vi "Deep Copy.vi"(8 "error in (no error)":errorcluster, 10 "Copy Actor In":refnum<class "System Actor.lvclass">, 11 "Root Actor in":refnum<class "Root Actor.lvclass">) -> (0 "error out":errorcluster, 2 "Coppied Actor Out":refnum<class "System Actor.lvclass">, 3 "Root Actor out":refnum<class "Root Actor.lvclass">)   [LabVIEW 2024, in "Root Actor.lvclass"]
uses:
  Root Actor.lvclass
  C:/Users/iio/Desktop/Bussiness/Tricorn Re/Madelbrot 4.0/General Library/Ancestor Class/Actor/System Actor/System Actor.lvclass
  System Actor/System Actor.lvclass
  Root Actor.lvclass/Root Actor.ctl
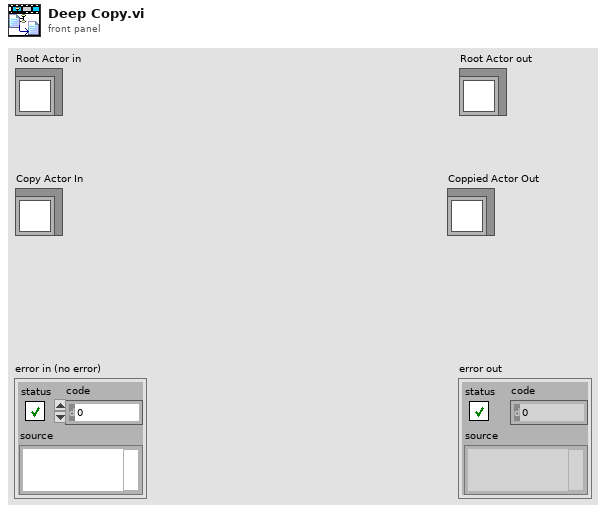
[diagram p1: front panel]
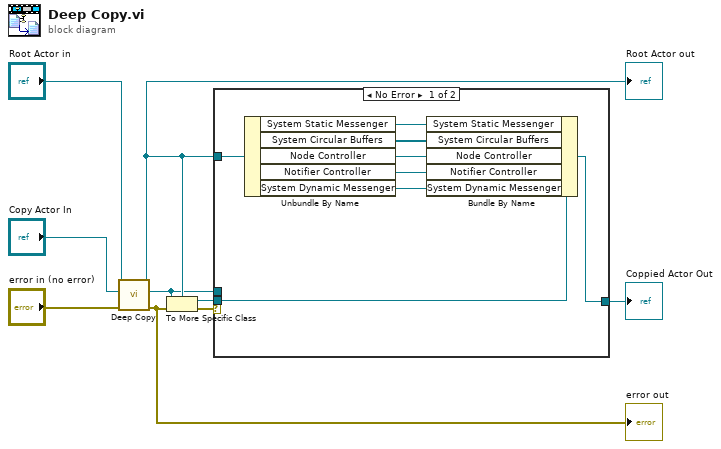
[diagram p0: block diagram]
diagram:
  n1 = call-parent "Deep Copy.vi"("error in (no error)"="error in (no error)", "Copy Actor In"="Copy Actor In", "System Actor in"="Root Actor in") -> ("error out"=w1:errorcluster, "Coppied Actor Out"=w2:refnum<class "System Actor.lvclass">, "System Actor out"=w6:refnum<class "Root Actor.lvclass">)  [unwired: 6 in]
  "error out" <- w1
  "Root Actor out" <- w6
  n2 = To More Specific Class(target class=w6, reference=w2, error in=w1) -> (specific class reference=w4:refnum<class "Root Actor.lvclass">, error out=w5:errorcluster)
  n3 = case shown="No Error" w5 {
    tunnel: w6 -> [w17 _]
    tunnel: w4 -> [w16 _]
    tunnel: [w10 w18] -> w3
    tunnel: w2 -> [_ w18]
    frame No Error {
      n4 = Unbundle By Name(w17) -> ("System Static Messenger"=w15:refnum<class "Messenger.lvclass">, "System Circular Buffers"=w14:refnum<class "Circular Buffer.lvclass">[], "Node Controller"=w13:refnum<class "Node Controller.lvclass">, "Notifier Controller"=w12:refnum<class "Notifier Controller.lvclass">, "System Dynamic Messenger"=w11:refnum<class "Messenger.lvclass">)
      n5 = Bundle By Name(cluster=w16, "System Static Messenger"=w15, "System Circular Buffers"=w14, "Node Controller"=w13, "Notifier Controller"=w12, "System Dynamic Messenger"=w11) -> (w10:refnum<class "Root Actor.lvclass">)
    }
    frame Error {
    }
  }
  "Coppied Actor Out" <- w3
